vi "Create LED Names_HE.vi"(0 "Expected LEDs":T1, 11 "Error In":errorcluster) -> (4 "Array of LED Names":string[](array[string]), 15 "Error Out":errorcluster)   [LabVIEW 2016, in "TLMB.lvlib"]
uses:
  Projects/TLMB.lvlib
  controls/HEUI_Display.ctl
  controls/Cycle Selection Enum.ctl
  controls/Stain Enum.ctl
  controls/Temp Enum.ctl
  controls/Soil Enum.ctl
  controls/Spin Enum.ctl
  controls/750 Status Enum.ctl
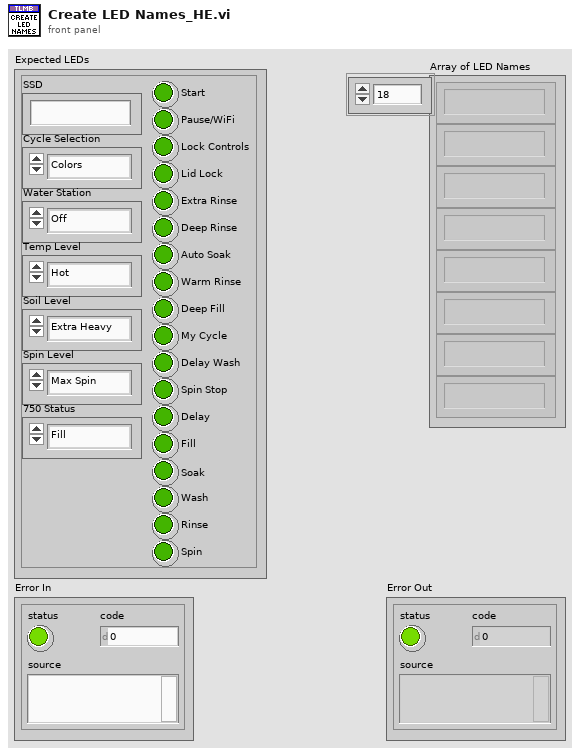
[diagram p1: front panel]
types:
  T1 = typedef "TLMB.lvlib/HEUI_Display.ctl" = cluster{"SSD":string, "Cycle Selection":T2, "Water Station":T3, "Temp Level":T4, "Soil Level":T5, "Spin Level":T6, "750 Status":T7, "Start":bool, "Pause/WiFi":bool, "Lock Controls":bool, "Lid Lock":bool, "Extra Rinse":bool, "Deep Rinse":bool, "Auto Soak":bool, "Warm Rinse":bool, "Deep Fill":bool, "My Cycle":bool, "Delay Wash":bool, "Spin Stop":bool, "Delay":bool, "Fill":bool, "Soak":bool, "Wash":bool, "Rinse":bool, "Spin":bool}
  T2 = typedef "TLMB.lvlib/Cycle Selection Enum.ctl" = enum16{"Colors", "Easy Care", "Delicates", "Hand Wash", "Active Wear", "Speed Wash", "Rinse and Spin", "Drain and Spin", "Basket Clean", "Jeans", "Heavy Duty", "Bulky Items", "Towels", "Whites", "Off", "*Incorrect*"}
  T3 = typedef "TLMB.lvlib/Stain Enum.ctl" = enum16{"Off", "Water", "Water & Detergent", "*Incorrect*"}
  T4 = typedef "TLMB.lvlib/Temp Enum.ctl" = enum16{"Hot", "Warm", "Colors", "Cool", "Cold", "Tap Cold", "Off", "*Incorrect*"}
  T5 = typedef "TLMB.lvlib/Soil Enum.ctl" = enum16{"Extra Heavy", "Heavy", "Normal", "Light", "Off", "*Incorrect*"}
  T6 = typedef "TLMB.lvlib/Spin Enum.ctl" = enum16{"Max Spin", "More Spin", "Normal Spin", "No Spin", "Off", "*Incorrect*"}
  T7 = typedef "TLMB.lvlib/750 Status Enum.ctl" = enum16{"Fill", "Wash", "Rinse", "Spin", "Off", "*Incorrect*"}
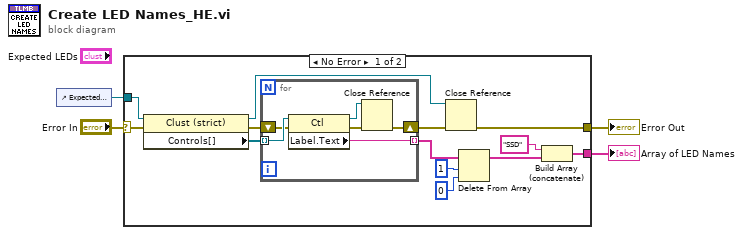
[diagram p0: block diagram]
diagram:
  n1 = control-ref of="Expected LEDs"() -> (w4:refnum<vi>)
  n2 = case shown="No Error" "Error In" {
    selector: "Error In" -> [w8 w24]
    tunnel: w4 -> [w17 _]
    tunnel: [w12 w24] -> w3
    tunnel: [w9 _] -> w2
    frame No Error {
      n3 = property class="Clust (strict)"(reference=w17, error in=w8) -> (reference out=w13:refnum<vi>, error out=w15:errorcluster, "Controls[]"=w16:refnum<vi>[])
      n4 = for {
        tunnel: w16 -> [w23] mode=indexing
        shift-right: [w19] -> w14
        shift-left: w15 -> [w22]
        tunnel: [w18] -> w7 mode=indexing
        n5 = property class="Ctl"(reference=w23, error in=w22) -> (reference out=w21:refnum<vi>, error out=w20:errorcluster, "Label.Text"=w18:string)
        n6 = Close Reference(reference=w21, error in (no error)=w20) -> (error out=w19:errorcluster)
      }
      n7 = Close Reference(reference=w13, error in (no error)=w14) -> (error out=w12:errorcluster)
      n8 = Delete From Array(array=w7, length=1, index=0) -> (array with subset deleted=w6:string[])  [unwired: 1 out]
      n9 = Build Array (concatenate)("SSD", w6) -> (w9:string[])
    }
    frame Error {
    }
  }
  "Error Out" <- w3
  "Array of LED Names" <- w2
